vi "FROG-GlobalVar.vi"() -> ()   [LabVIEW 2014]
doc: "Mapa de Intensidade FROG\n\nAndré Romero - 2022\nandretec@ifsc.usp.br"
panel:
  out "GO":bool
  out "Tipo":bool
  in  "Progresso":i32
  # "False -> 1 Linha por ciclo\nTrue  -> 2 Linhas por ciclo"
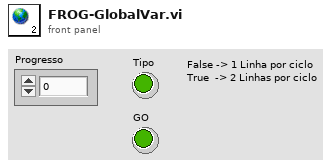
[diagram p1: front panel]
diagram:
